vi "量程参数设置.vi"(10 "自动测试量程配置":T5={"水样测试量程模式"=enum."H", "标样核查量程模式"=enum."H", "零点核查量程模式"=enum."H", "跨度核查量程模式"=enum."H", "空白测试量程模式"=enum."H", "平行样测试量程模式"=enum."H", "加标回收量程模式"=enum."H", "空白校准量程模式"=enum."H", "标样校准量程模式"=enum."H"}, 11 "质控参数设置":T4) -> (1 "checkout":bool, 2 "自动测试量程配置 2":T2={"水样测试量程模式"=enum."H", "标样核查量程模式"=enum."H", "零点核查量程模式"=enum."H", "跨度核查量程模式"=enum."H", "空白测试量程模式"=enum."H", "平行样测试量程模式"=enum."H", "加标回收量程模式"=enum."H", "标样校准量程模式"=enum."H", "空白校准量程模式"=enum."H"}, 3 "输出簇":T3)   [LabVIEW 2016]
uses:
  <vilib>/Utility/miscctls.llb/LVPointTypeDef.ctl
panel:
  in  "codmn标准液标准浓度":dbl
  in  "codmn跨度标准液浓度":dbl
  in  "codmn零点标准液浓度":dbl
  in  "codmn跨度值":dbl
  in  "取消":bool
  in  "确定":bool
  # "量程、质控参数设置"
  # "质控上传平台参数设置"
  # "跨度值"
  # "mg/L"
  # "零点核查标准液浓度"
  # "mg/L"
  # "跨度核查标准液浓度"
  # "mg/L"
  # "标样核查标准液浓度"
  # "mg/L"
  # "质控参数设置"
  # "监测参数"
  # "codmn"
  # "跨度值"
  # "零点核查标准液浓度"
  # "跨度核查标准液浓度"
  # "标样核查标准液浓度"
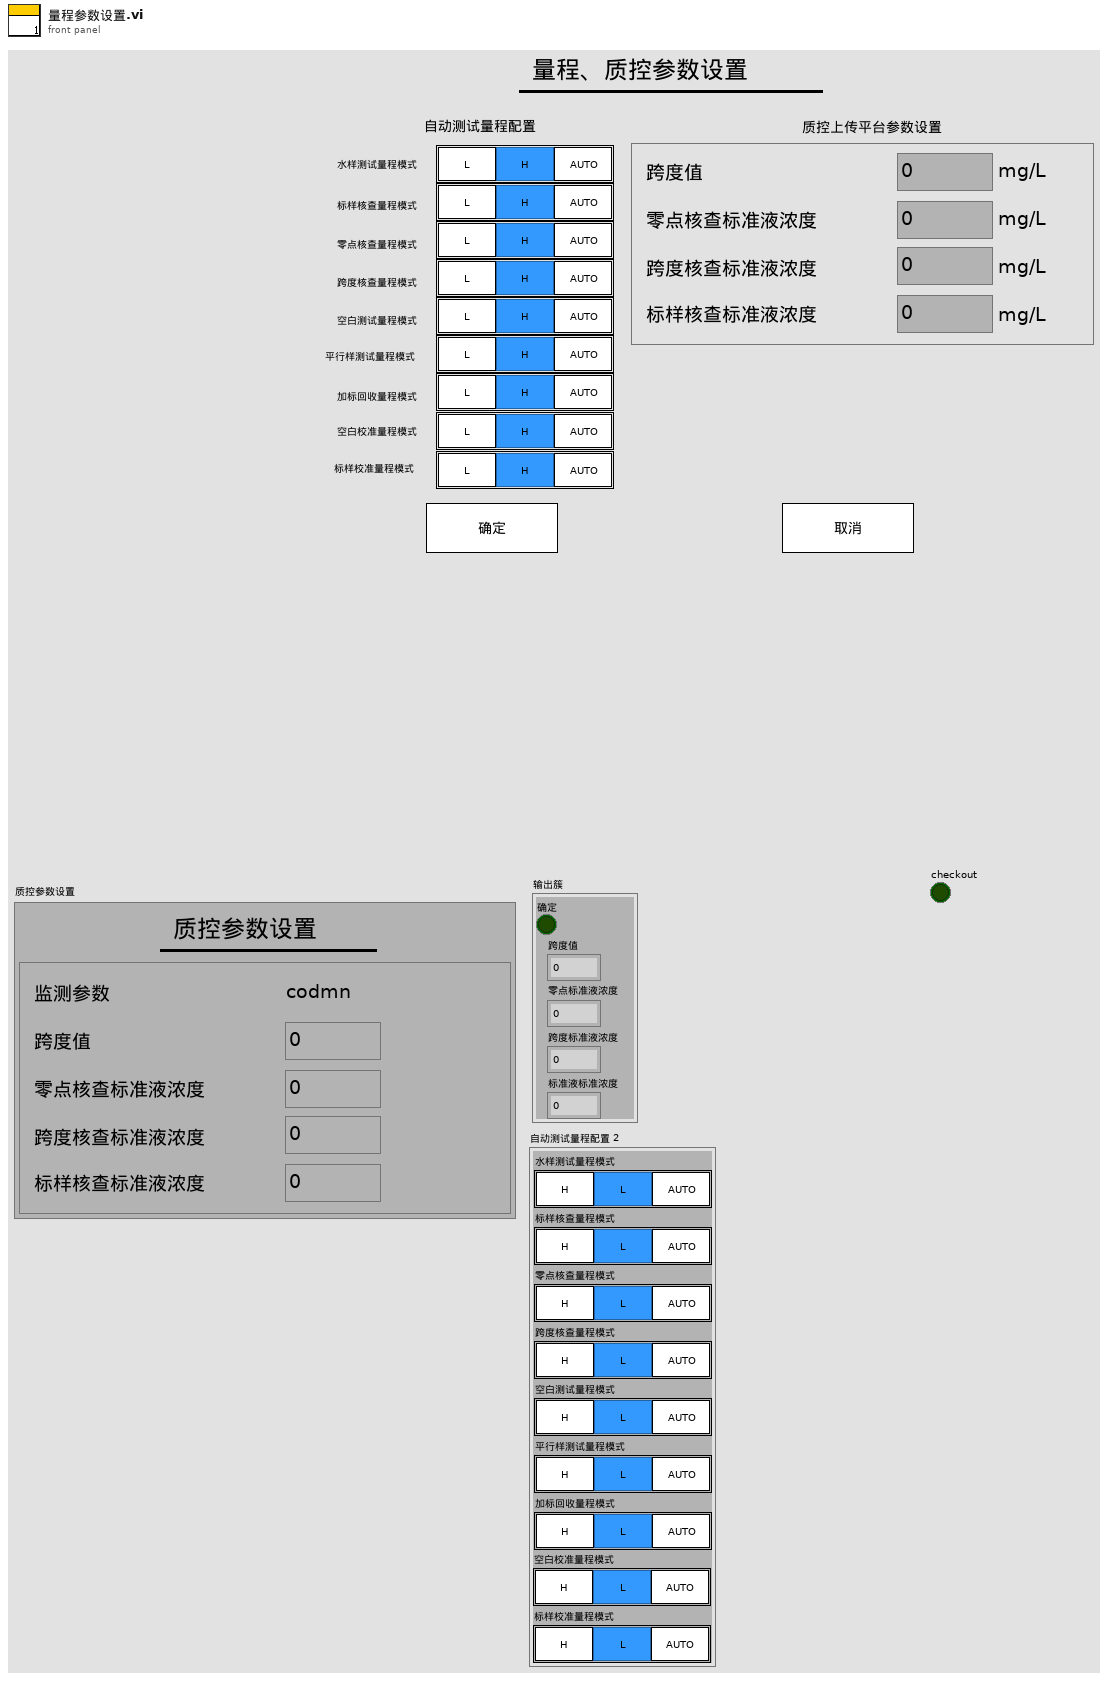
[diagram p1: front panel]
types:
  T1 = typedef "量程选择控件.ctl" = enum32{"L", "H", "AUTO"}
  T2 = cluster{"水样测试量程模式":T1, "标样核查量程模式":T1, "零点核查量程模式":T1, "跨度核查量程模式":T1, "空白测试量程模式":T1, "平行样测试量程模式":T1, "加标回收量程模式":T1, "标样校准量程模式":T1, "空白校准量程模式":T1}
  T3 = cluster{"确定":bool, "跨度值":dbl, "零点标准液浓度":dbl, "跨度标准液浓度":dbl, "标准液标准浓度":dbl}
  T4 = cluster{"总磷跨度值":dbl, "总磷零点标准液浓度":dbl, "总磷跨度标准液浓度":dbl, "总磷标准液标准浓度":dbl}
  T5 = cluster{"水样测试量程模式":T1, "标样核查量程模式":T1, "零点核查量程模式":T1, "跨度核查量程模式":T1, "空白测试量程模式":T1, "平行样测试量程模式":T1, "加标回收量程模式":T1, "空白校准量程模式":T1, "标样校准量程模式":T1}
  T6 = typedef "LVPointTypeDef.ctl" = cluster{"Horizontal":i16, "Vertical":i16}
  T7 = cluster{"确定":bool, "codmn跨度值":dbl, "codmn零点标准液浓度":dbl, "codmn跨度标准液浓度":dbl, "codmn标准液标准浓度":dbl}
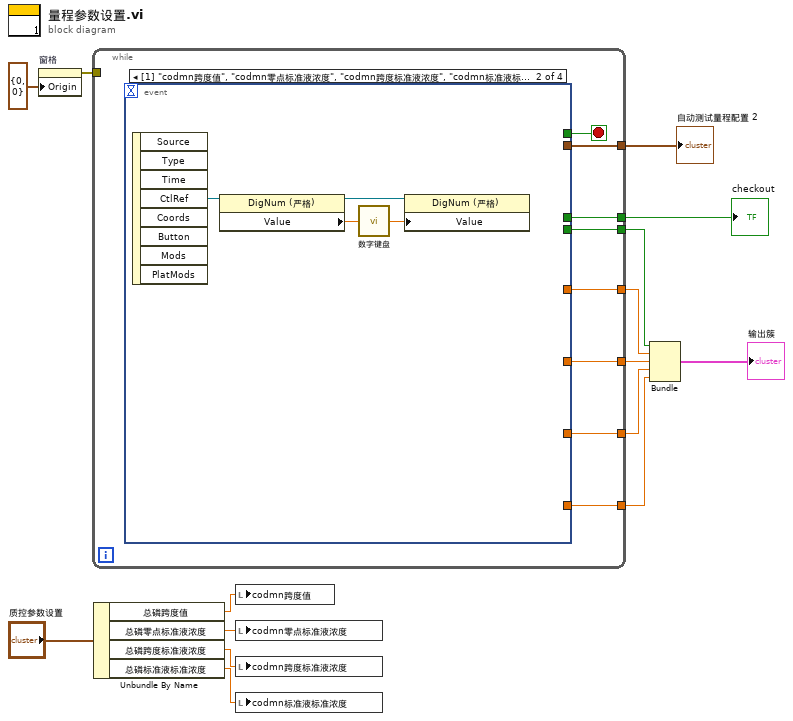
[diagram p0: block diagram]
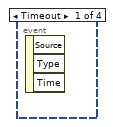
[diagram p2: hidden frame]
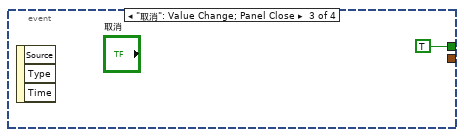
[diagram p3: hidden frame]
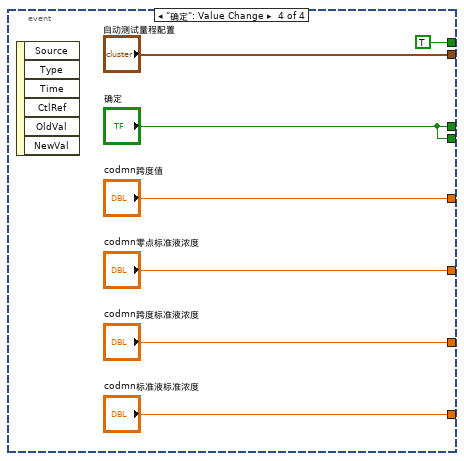
[diagram p4: hidden frame]
diagram:
  n1 = property on="窗格" class="Pane"("Origin"=T6 {"Horizontal"=0, "Vertical"=0} ("原点")) -> (error out=w14:errorcluster)  [unwired: 2 in, 1 out]
  n2 = while {
    tunnel: w14 -> [_]
    tunnel: [w22] -> w13
    tunnel: [w21] -> w1
    tunnel: [w20] -> w7
    tunnel: [w19] -> w6
    tunnel: [w18] -> w5
    tunnel: [w17] -> w4
    tunnel: [w16] -> w3
    stop <- w23 stop-if-true
    n3 = event shown="[1] \"codmn跨度值\", \"codmn零点标准液浓度\", \"codmn跨度标准液浓度\", \"codmn标准液标准浓度\": 鼠标按下" {
      selector: _ -> [_ _ _ _]
      dyn-events: _ -> [_ _ _ _]
      timeout: _ -> [_ _ _ _]
      tunnel: [_ _ TRUE TRUE] -> w23
      tunnel: [_ _ _ "确定"] -> w22
      tunnel: [_ _ _ "自动测试量程配置"] -> w21
      tunnel: [_ _ _ "确定"] -> w20
      tunnel: [_ _ _ "codmn跨度值"] -> w19
      tunnel: [_ _ _ "codmn零点标准液浓度"] -> w18
      tunnel: [_ _ _ "codmn跨度标准液浓度"] -> w17
      tunnel: [_ _ _ "codmn标准液标准浓度"] -> w16
      event Timeout {
        n4 = event-data() -> ()  [unwired: 1 in, 3 out]
      }
      event "codmn跨度值", "codmn零点标准液浓度", "codmn跨度标准液浓度", "codmn标准液标准浓度": Mouse Down {
        n5 = event-data() -> ("CtlRef"=w24:refnum<vi>)  [unwired: 1 in, 7 out]
        n6 = property class="DigNum (严格)"(reference=w24) -> (reference out=w27:refnum<vi>, "Value"=w26:dbl)  [unwired: 1 in, 1 out]
        n7 = call "数字键盘.vi"("OldNumber"=w26) -> ("NewNumber"=w25:dbl)
        n8 = property class="DigNum (严格)"(reference=w27, "Value"=w25) -> ()  [unwired: 1 in, 2 out]
      }
      event "取消": Value Change; Panel Close {
        n9 = event-data() -> ()  [unwired: 1 in, 3 out]
      }
      event "确定": Value Change {
        n10 = event-data() -> ()  [unwired: 1 in, 6 out]
      }
    }
  }
  "checkout" <- w13
  "自动测试量程配置 2" <- w1
  n11 = Unbundle By Name("质控参数设置") -> ("总磷跨度值"=w11:dbl, "总磷零点标准液浓度"=w10:dbl, "总磷跨度标准液浓度"=w9:dbl, "总磷标准液标准浓度"=w8:dbl)
  n12 = local write "codmn跨度值"(w11) -> ()
  n13 = local write "codmn零点标准液浓度"(w10) -> ()
  n14 = local write "codmn跨度标准液浓度"(w9) -> ()
  n15 = local write "codmn标准液标准浓度"(w8) -> ()
  n16 = Bundle("确定"=w7, "codmn跨度值"=w6, "codmn零点标准液浓度"=w5, "codmn跨度标准液浓度"=w4, "codmn标准液标准浓度"=w3) -> (→"输出簇":T7)  [unwired: 1 in]
